vi "运维调试_五参数.vi"() -> ()   [LabVIEW 2016, in "斯坦道仪器.lvlib"]
uses:
  <vilib>/Utility/miscctls.llb/LVPointTypeDef.ctl
  PLC/PLC.lvlib
panel:
  in  "打开串口":bool
  in  "释放串口":bool
  in  "手动通电":bool
  out "多参数横条运行状态":T1(xcontrol)
  in  "数据区":i32(listbox)
  in  "探头选择":u16(ring)=9 items=["氨氮"=3, "水温"=9, "pH值"=10, "溶解氧"=11, "电导率"=12, "浊度"=13, "叶绿素a"=14, "藻密度"=15, "蓝绿藻"=16, "氧化还原电位"=17, "溶解氧%"=18, "盐度"=19]
  in  "测量数据区读取":bool
  in  "测量数据区":i32(listbox)
  in  "状态告警区读取":bool
  in  "状态告警区":i32(listbox)
  in  "自动校准":bool
  in  "读取KB":bool
  in  "写入KB":bool
  out "B":dbl caption="校准值B:"
  out "K":dbl caption="校准值K:"
  in  "校准区探头选择":u16(ring)=9 items=["氨氮"=3, "水温"=9, "pH值"=10, "溶解氧"=11, "电导率"=12, "浊度"=13, "叶绿素a"=14, "藻密度"=15, "蓝绿藻"=16, "氧化还原电位"=17, "溶解氧%"=18, "盐度"=19]
  in  "停止测量(单探)":bool
  in  "启动测量(单探)":bool
  in  "控制命令区探头选择":u16(ring)=9 items=["氨氮"=3, "水温"=9, "pH值"=10, "溶解氧"=11, "电导率"=12, "浊度"=13, "叶绿素a"=14, "藻密度"=15, "蓝绿藻"=16, "氧化还原电位"=17, "溶解氧%"=18, "盐度"=19]
  in  "同步时间":bool
  in  "初始化(清洗)":bool
  in  "停止测量(全部)":bool
  in  "启动测量(全部)":bool
  in  "关键参数区读取":bool
  in  "关键参数区":i32(listbox)
  in  "传感器参数读取":bool
  in  "传感器区":i32(listbox)
  in  "返回":bool
  in  "设置":bool
  out "运行状态":string
  out "开机状态":bool
  in  "停止":bool
  in  "手动启动":bool
  out "集成报警信息":string
  # "控制命令区"
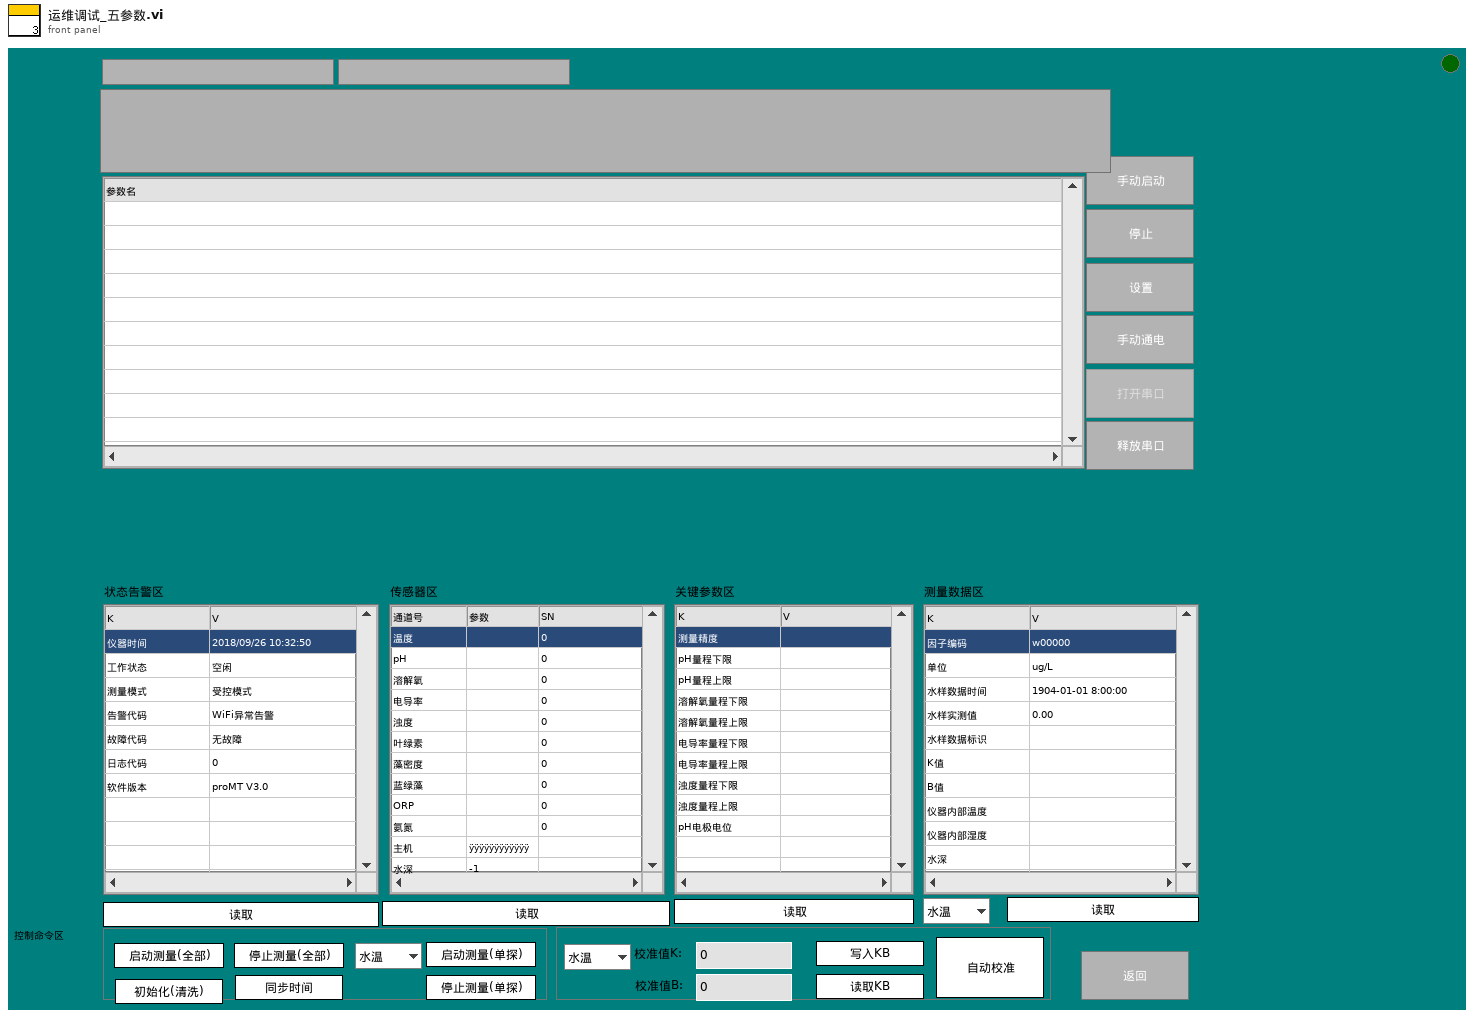
[diagram p1: front panel]
types:
  T1 = cluster{"系统时间":timestamp, "工作状态":u16, "测量模式":u16, "告警代码":enum16{"无告警", "缺试剂告警", "缺水样告警", "缺蒸馏水告警", "缺标液告警", "仪表漏液告警", "标定异常告警", "超量程告警", "加热异常", "低试剂预警", "超上限告警", "超下限告警", "仪表内部其他异常", "滴定异常告警", "电极异常告警", "量程切换告警", "参数设置告警", "PH电极电位异常", "电导率电极异常", "浊度光度异常", "溶解氧电极异常", "溶解氧光强异常", "温度异常告警", "PH异常告警", "溶解氧异常告警", "电导率异常告警", "浊度异常告警", "叶绿素异常告警", "藻密度异常告警", "蓝绿藻异常告警", "ORP异常告警", "氨氮异常告警", "清洁刷异常告警", "SD卡异常告警", "蓝牙异常告警", "Wifi异常告警", "流程异常告警"}, "故障代码":enum16{"无故障", "电机故障", "温度故障", "通讯故障", "滴定故障"}, "日志代码":u16, "软件版本":string}
  T2 = typedef "LVPointTypeDef.ctl" = cluster{"Horizontal":i16, "Vertical":i16}
  T3 = cluster{"时间标识":timestamp, "设备":string, "日志信息":string}
  T4 = enum16{"无告警", "缺试剂告警", "缺水样告警", "缺蒸馏水告警", "缺标液告警", "仪表漏液告警", "标定异常告警", "超量程告警", "加热异常", "低试剂预警", "超上限告警", "超下限告警", "仪表内部其他异常", "滴定异常告警", "电极异常告警", "量程切换告警", "参数设置告警", "PH电极电位异常", "电导率电极异常", "浊度光度异常", "溶解氧电极异常", "溶解氧光强异常", "温度异常告警", "PH异常告警", "溶解氧异常告警", "电导率异常告警", "浊度异常告警", "叶绿素异常告警", "藻密度异常告警", "蓝绿藻异常告警", "ORP异常告警", "氨氮异常告警", "清洁刷异常告警", "SD卡异常告警", "蓝牙异常告警", "Wifi异常告警", "流程异常告警"}
  T5 = cluster{"水温":dbl, "pH":dbl, "DO":dbl, "Cond":dbl, "Turb":dbl, "叶绿素":dbl, "藻密度":dbl, "蓝绿藻":dbl, "ORP":dbl, "NH3N":dbl}
  T6 = cluster{"因子编码":string, "单位":string, "标样参考值":sgl, "水样数据时间":timestamp, "水样实测值":sgl, "水样数据标识":string, "K":sgl, "B":sgl, "T":sgl, "H":sgl, "水深":sgl}
  T7 = enum8{"Enabled", "Disabled", "Disabled and Grayed Out"}
  T8 = cluster{"测量模式":enum16{"待机", "水样测试", "标样核查", "零点核查", "跨度核查", "空白测试", "平行样测试", "加标回收", "空白校准", "标样校准", "初始化（清洗）"}, "数据标记表":string, "测量时间":dbl}
  T9 = cluster{"starting address":u16, "holding register value":u16}
  T10 = enum16{"idle", "init", "读状态", "读参数", "多个写入", "单个写入", "线圈写入"}
  T11 = enum32{"Bad", "Idle", "Run top level", "Running"}
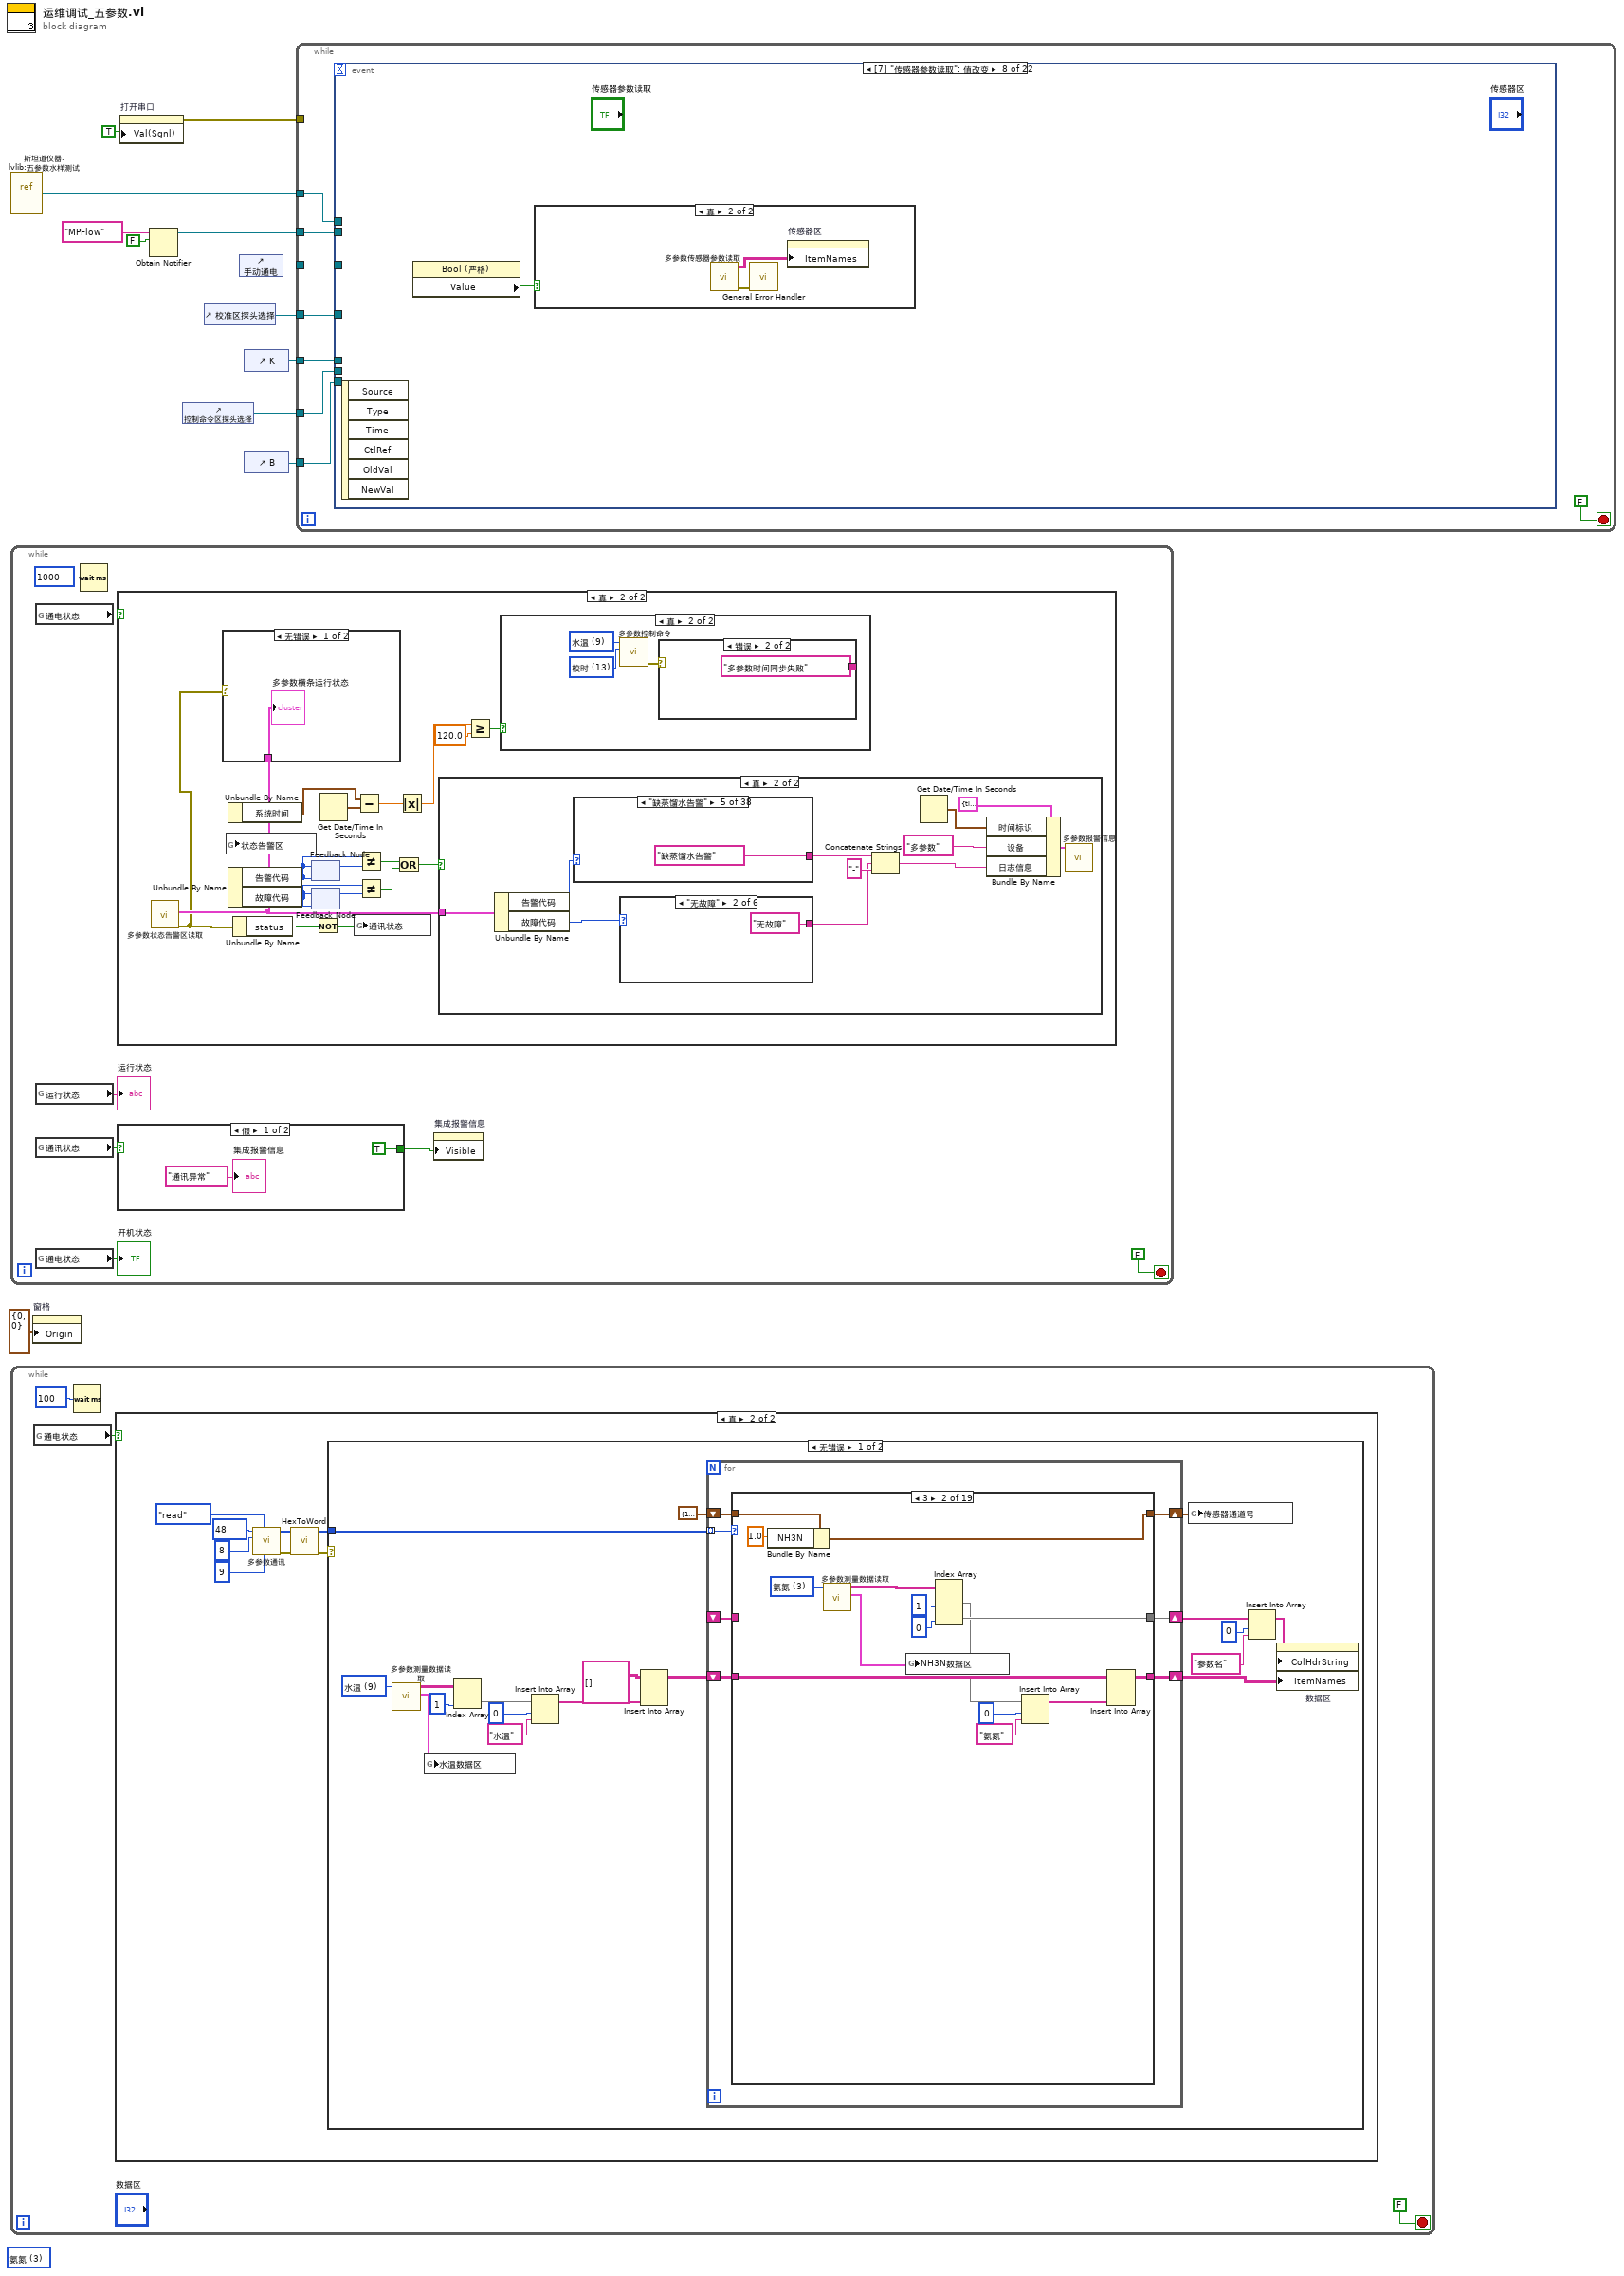
[diagram p0: block diagram]
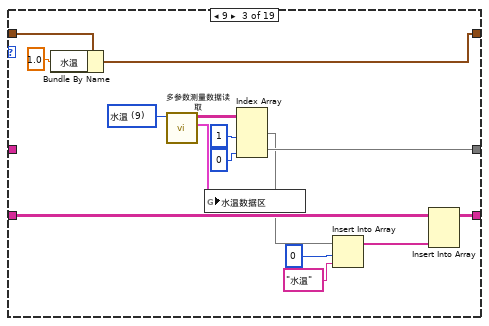
[diagram p4: hidden frame]
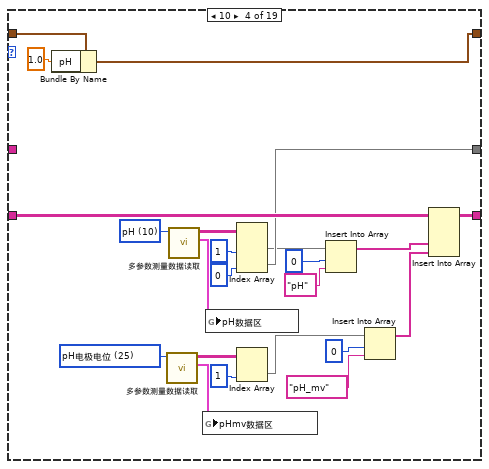
[diagram p5: hidden frame]
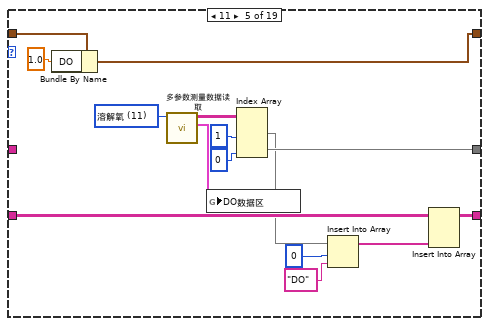
[diagram p6: hidden frame]
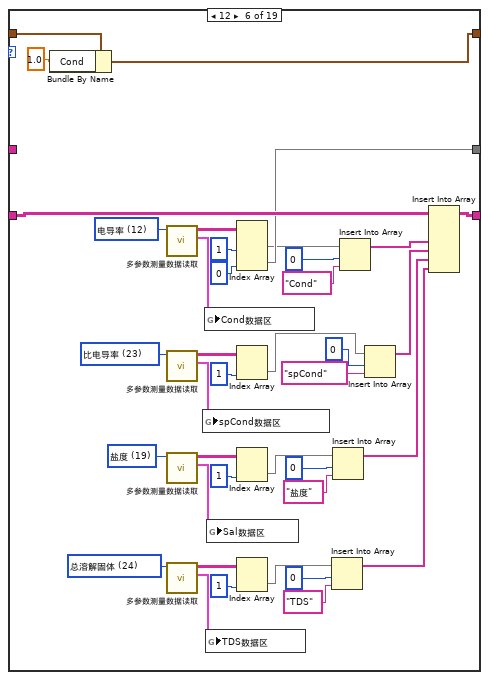
[diagram p7: hidden frame]
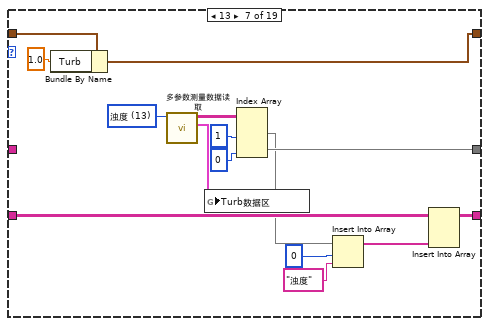
[diagram p8: hidden frame]
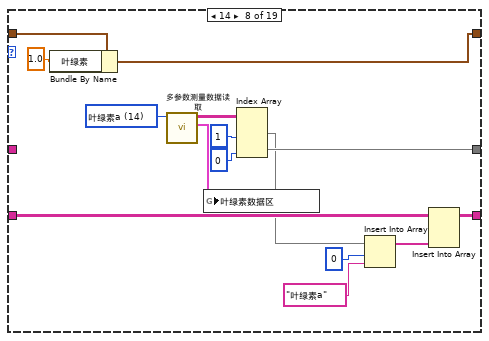
[diagram p9: hidden frame]
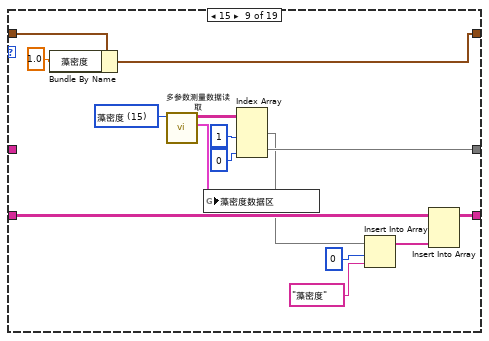
[diagram p10: hidden frame]
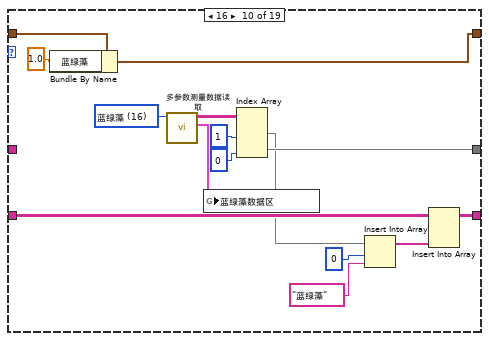
[diagram p11: hidden frame]
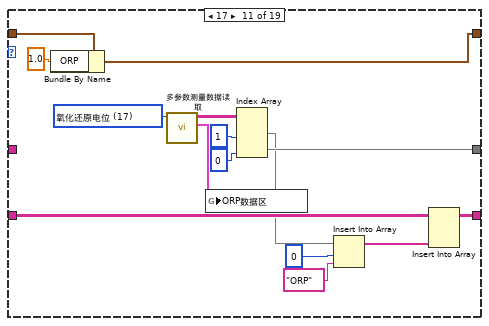
[diagram p12: hidden frame]
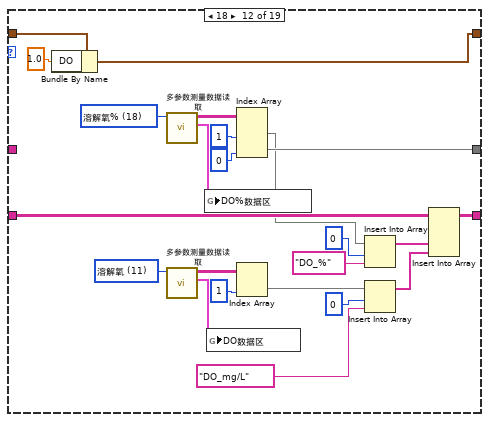
[diagram p13: hidden frame]
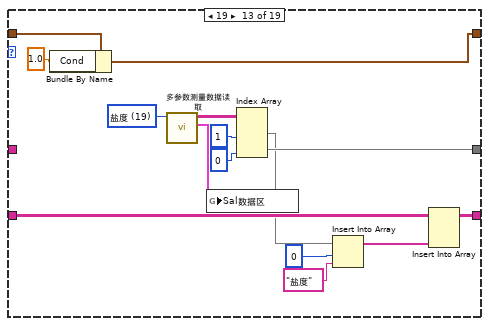
[diagram p14: hidden frame]
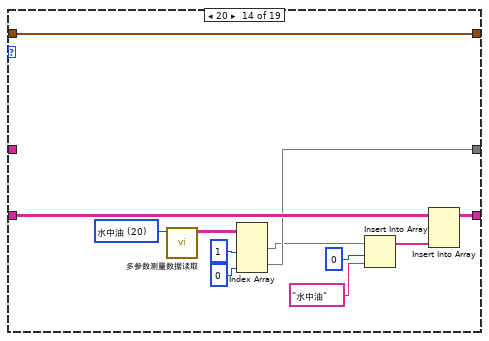
[diagram p15: hidden frame]
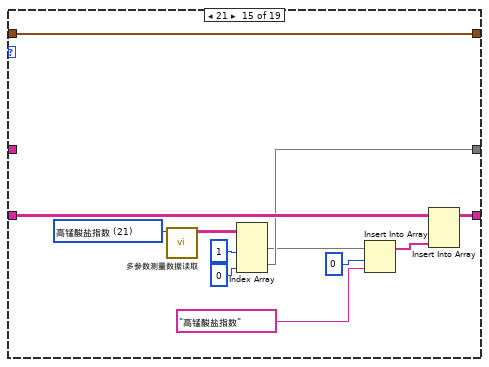
[diagram p16: hidden frame]
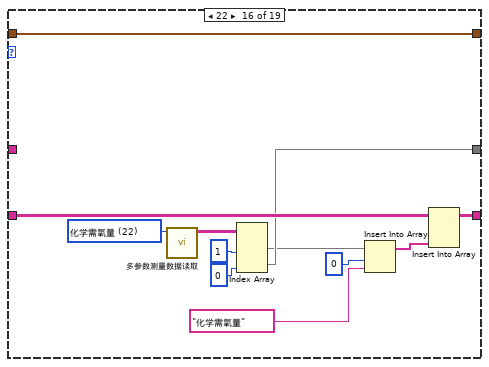
[diagram p17: hidden frame]
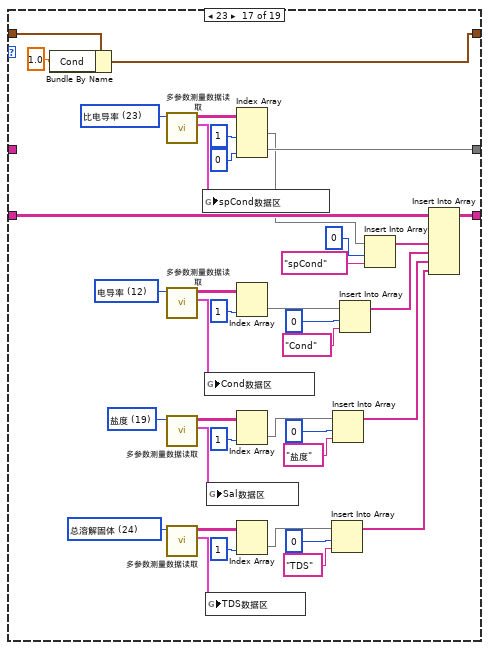
[diagram p18: hidden frame]
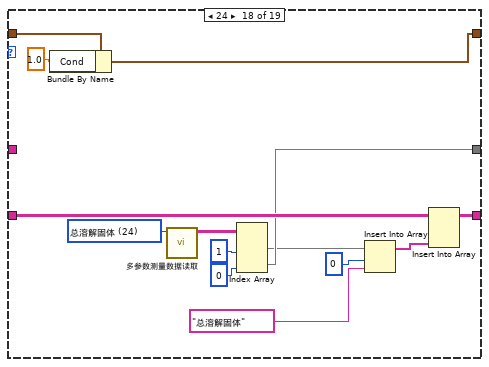
[diagram p19: hidden frame]
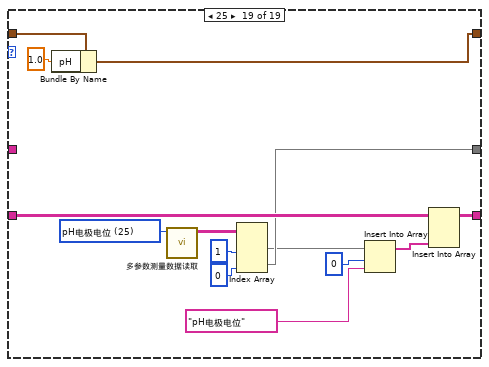
[diagram p20: hidden frame]
diagram:
  (unwired) u16 3 items=["氨氮"=3, "水温"=9, "pH"=10, "溶解氧"=11, "电导率"=12, "浊度"=13, "叶绿素a"=14, "藻密度"=15, "蓝绿藻"=16, "氧化还原电位"=17, "溶解氧%"=18, "盐度"=19, "水中油"=20, "高锰酸盐指数"=21, "化学需氧量"=22, "比电导率"=23, "总溶解固体"=24, "pH电极电位"=25] ("下拉列表")
  n1 = vi-ref "斯坦道仪器.lvlib:五参数水样测试.vi"() -> (w9:refnum<vi>)
  n2 = while {
    stop <- FALSE stop-if-true
    n3 = global read "多参数全局变量.vi" "通电状态"() -> (w13:bool)
    n4 = global read "多参数全局变量.vi" "运行状态"() -> (→"运行状态":string)
    n5 = global read "多参数全局变量.vi" "通讯状态"() -> (w17:bool)
    n6 = global read "多参数全局变量.vi" "通电状态"() -> (→"开机状态":bool)
    n7 = Wait (ms)(milliseconds to wait=u32 1000 ("等待时间（毫秒）")) -> ()  [unwired: 1 out]
    n8 = case shown="真" w13 {
      frame False {
      }
      frame True {
        n9 = call "多参数状态告警区读取.vi"() -> ("error out"=w20:errorcluster, "状态告警块"=w27:T1)  [unwired: 9 in, 1 out]
        n10 = case shown="无错误" w20 {
          tunnel: w27 -> [w37 _]
          frame No Error {
            "多参数横条运行状态" <- w37
          }
          frame Error {
          }
        }
        n11 = global write "多参数全局变量.vi" "状态告警区"(w27) -> ()
        n12 = Unbundle By Name(w27) -> ("系统时间"=w26:timestamp)
        n13 = Unbundle By Name(w27) -> ("告警代码"=w35:T4, "故障代码"=w33:enum16{"无故障", "电机故障", "温度故障", "通讯故障", "滴定故障"})
        n14 = Unbundle By Name(w20) -> ("status"=w29:bool)
        n15 = feedback #1(w35) -> (w36:T4)
        n16 = feedback-in #1(w35) -> ()
        n17 = feedback #2(w33) -> (w34:enum16{"无故障", "电机故障", "温度故障", "通讯故障", "滴定故障"})
        n18 = feedback-in #2(w33) -> ()
        n19 = Not(x=w29) -> (.not. x?=w28:bool)
        n20 = Get Date/Time In Seconds() -> (seconds since 1Jan1904=w25:timestamp)
        n21 = global write "多参数全局变量.vi" "通讯状态"(w28) -> ()
        n22 = Subtract(x=w26, y=w25) -> (x-y=w24:dbl)
        n23 = Not Equal?(x=w35, y=w36) -> (x != y?=w31:bool)
        n24 = Not Equal?(x=w33, y=w34) -> (x != y?=w32:bool)
        n25 = Or(x=w31, y=w32) -> (x .or. y?=w30:bool)
        n26 = Absolute Value(x=w24) -> (abs(x)=w23:dbl)
        n27 = case shown="真" w30 {
          tunnel: w27 -> [_ w53]
          frame False {
          }
          frame True {
            n28 = Unbundle By Name(w53) -> ("告警代码"=w52:T4, "故障代码"=w51:enum16{"无故障", "电机故障", "温度故障", "通讯故障", "滴定故障"})
            n29 = case shown="\"缺蒸馏水告警\"" w52 {
              selector: w52 -> [w64 _ _ _ _ _ _ _ _ _ _ _ _ _ _ _ _ _ _ _ _ _ _ _ _ _ _ _ _ _ _ _ _ _ _ _ _ _]
              tunnel: [w63 "无告警" "缺试剂告警" "缺水样告警" "缺蒸馏水告警" "缺标液告警" "仪表漏液告警" "标定异常告警" "超量程告警" "加热异常" "低试剂预警" "超上限告警" "超下限告警" "仪表内部其他异常" "滴定异常告警" "电极异常告警" "量程切换告警" "参数设置告警" "PH电极电位异常" "电导率电极异常" "浊度光度异常" "溶解氧电极异常" "溶解氧光强异常" "温度异常告警" "PH异常告警" "溶解氧异常告警" "电导率异常告警" "浊度异常告警" "叶绿素异常告警" "藻密度异常告警" "蓝绿藻异常告警" "ORP异常告警" "氨氮异常告警" "清洁刷异常告警" "SD卡异常告警" "蓝牙异常告警" "WiFi异常告警" "流程异常告警"] -> w50
              frame Default {
                n30 = Format Into String(format string="%d" ("格式字符串"), initial string="未知" ("工作状态"), w64) -> (resulting string=w63:string)  [unwired: 1 in, 1 out]
              }
              frame "无告警" {
              }
              frame "缺试剂告警" {
              }
              frame "缺水样告警" {
              }
              frame "缺蒸馏水告警" {
              }
              frame "缺标液告警" {
              }
              frame "仪表漏液告警" {
              }
              frame "标定异常告警" {
              }
              frame "超量程告警" {
              }
              frame "加热异常" {
              }
              frame "低试剂预警" {
              }
              frame "超上限告警" {
              }
              frame "超下限告警" {
              }
              frame "仪表内部其他异常" {
              }
              frame "滴定异常告警" {
              }
              frame "电极异常告警" {
              }
              frame "量程切换告警" {
              }
              frame "参数设置告警" {
              }
              frame "PH电极电位异常" {
              }
              frame "电导率电极异常" {
              }
              frame "浊度光度异常" {
              }
              frame "溶解氧电极异常" {
              }
              frame "溶解氧光强异常" {
              }
              frame "温度异常告警" {
              }
              frame "PH异常告警" {
              }
              frame "溶解氧异常告警" {
              }
              frame "电导率异常告警" {
              }
              frame "浊度异常告警" {
              }
              frame "叶绿素异常告警" {
              }
              frame "藻密度异常告警" {
              }
              frame "蓝绿藻异常告警" {
              }
              frame "ORP异常告警" {
              }
              frame "氨氮异常告警" {
              }
              frame "清洁刷异常告警" {
              }
              frame "SD卡异常告警" {
              }
              frame "蓝牙异常告警" {
              }
              frame "Wifi异常告警" {
              }
              frame "流程异常告警" {
              }
            }
            n31 = case shown="\"无故障\"" w51 {
              selector: w51 -> [w55 _ _ _ _ _]
              tunnel: [w54 "无故障" "电机故障" "温度故障" "通讯故障" "滴定故障"] -> w49
              frame Default {
                n32 = Format Into String(format string="%d" ("格式字符串"), initial string="未知" ("工作状态"), w55) -> (resulting string=w54:string)  [unwired: 1 in, 1 out]
              }
              frame "无故障" {
              }
              frame "电机故障" {
              }
              frame "温度故障" {
              }
              frame "通讯故障" {
              }
              frame "滴定故障" {
              }
            }
            n33 = Concatenate Strings(w50, "-" ("字符串"), w49) -> (w45:string)
            n34 = Get Date/Time In Seconds() -> (seconds since 1Jan1904=w44:timestamp)
            n35 = Bundle By Name(cluster=T3 {"时间标识"=timestamp(0 s since 1904-01-01), "设备"="", "日志信息"=""} ("data in"), "时间标识"=w44, "设备"="多参数", "日志信息"=w45) -> (w46:T3)
            n36 = call "多参数报警信息.vi"("data in"=w46) -> ()  [unwired: 10 in, 1 out]
          }
        }
        n37 = Greater Or Equal?(x=w23, y=120.0) -> (x >= y?=w22:bool)
        n38 = case shown="真" w22 {
          frame False {
          }
          frame True {
            w38 = u16 13 items=["启动测量（全部）"=1, "初始化（清洗）"=10, "停止测量（全部）"=11, "校时"=13, "启动测量（单个传感器）"=19, "停止测量（单个传感器）"=20] ("控制命令")
            w39 = u16 9 items=["氨氮"=3, "水温"=9, "pH值"=10, "溶解氧"=11, "电导率"=12, "浊度"=13, "叶绿素a"=14, "藻密度"=15, "蓝绿藻"=16, "氧化还原电位"=17, "溶解氧%"=18, "盐度"=19] ("站号")
            n39 = call "多参数控制命令.vi"("控制命令"=w38, "站号"=w39) -> ("error out"=w40:errorcluster)  [unwired: 9 in]
            n40 = case shown="错误" w40 {
              tunnel: ["多参数时间同步成功" ("消息") "多参数时间同步失败" ("消息")] -> _
              frame No Error {
              }
              frame Error {
              }
            }
          }
        }
      }
    }
    n41 = case shown="假" w17 {
      tunnel: [TRUE ("可见") _] -> w16
      frame False {
        "集成报警信息" <- "通讯异常" ("集成报警信息")
      }
      frame True {
      }
    }
    n42 = property on="集成报警信息" class="Str"("Visible"=w16) -> ()  [unwired: 2 in, 2 out]
  }
  n43 = while {
    stop <- FALSE stop-if-true
    n44 = global read "多参数全局变量.vi" "通电状态"() -> (w106:bool)
    n45 = Wait (ms)(milliseconds to wait=u32 100 ("等待时间（毫秒）")) -> ()  [unwired: 1 out]
    n46 = case shown="真" w106 {
      frame False {
      }
      frame True {
        n47 = call "多参数通讯.vi"("Slave ID"=u8 9, "STEP"=enum16{"open", "read", "write", "close"}."read", "quantity"=u16 8, "starting address"=u16 48) -> ("error out"=w111:errorcluster, "Registers"=w112:u16[])  [unwired: 5 in, 1 out]
        n48 = call "HexToWord.vi"("数组"=w112) -> ("WORD"=w115:u16[])  [unwired: 10 in]
        n49 = case shown="无错误" w111 {
          tunnel: w115 -> [w130 _]
          frame No Error {
            w127 = u16 9 items=["氨氮"=3, "水温"=9, "pH"=10, "溶解氧"=11, "电导率"=12, "浊度"=13, "叶绿素a"=14, "藻密度"=15, "蓝绿藻"=16, "氧化还原电位"=17, "溶解氧%"=18, "盐度"=19, "水中油"=20, "高锰酸盐指数"=21, "化学需氧量"=22, "比电导率"=23, "总溶解固体"=24, "pH电极电位"=25] ("下拉列表")
            n50 = call "多参数测量数据读取.vi"("探头选择"=w127) -> ("测量数据块"=w116:T6, "添加的数组"=w126:string[][])  [unwired: 8 in, 1 out]
            n51 = global write "多参数全局变量.vi" "水温数据区"(w116) -> ()
            n52 = Index Array(array=w126, index (col)=1 ("禁用的索引 (列)")) -> (element=w121:string[])  [unwired: 1 in]
            n53 = Insert Into Array(array=w121, index=0 ("索引"), new element="水温") -> (w123:string[])
            n54 = Insert Into Array(array=string[][] [] ("子数组"), new element=w123) -> (w119:string[][])  [unwired: 2 in]
            n55 = for {
              tunnel: w130 -> [w140] mode=indexing
              shift-right: [w138] -> w128
              shift-left: w119 -> [w139]
              shift-right: [w137] -> w129
              shift-left: _ -> [w136]
              shift-right: [w135] -> w117
              shift-left: T5 {"水温"=1.0, "pH"=0.0, "DO"=0.0, "Cond"=0.0, "Turb"=0.0, "叶绿素"=0.0, "藻密度"=0.0, "蓝绿藻"=0.0, "ORP"=0.0, "NH3N"=0.0} ("传感器通道号") -> [w134]
              n56 = case shown="3" w140 {
                tunnel: w139 -> [w143 w154 w169 w192 w207 w246 w261 w276 w291 w306 w321 w344 w359 w371 w383 w395 w434 w448 w462]
                tunnel: [w143 w153 w168 w191 w206 w245 w260 w275 w290 w305 w320 w343 w358 w370 w382 w394 w433 w447 w461] -> w138
                tunnel: [w142 w151 w166 w189 w204 w243 w258 w273 w288 w303 w318 w341 w356 w368 w380 w392 w431 w445 w459] -> w137
                tunnel: w136 -> [w142 _ _ _ _ _ _ _ _ _ _ _ _ _ _ _ _ _ _]
                tunnel: [w141 w145 w160 w176 w198 w216 w252 w267 w282 w297 w312 w328 w350 w364 w376 w388 w425 w439 w453] -> w135
                tunnel: w134 -> [w141 w147 w162 w178 w200 w217 w253 w268 w283 w298 w313 w329 w351 w364 w376 w388 w426 w440 w454]
                frame 0, Default {
                }
                frame 3 {
                  w158 = u16 3 items=["氨氮"=3, "水温"=9, "pH"=10, "溶解氧"=11, "电导率"=12, "浊度"=13, "叶绿素a"=14, "藻密度"=15, "蓝绿藻"=16, "氧化还原电位"=17, "溶解氧%"=18, "盐度"=19, "水中油"=20, "高锰酸盐指数"=21, "化学需氧量"=22, "比电导率"=23, "总溶解固体"=24, "pH电极电位"=25] ("下拉列表")
                  n57 = Bundle By Name(cluster=w147, "NH3N"=1.0) -> (w145:T5)
                  n58 = call "多参数测量数据读取.vi"("探头选择"=w158) -> ("测量数据块"=w144:T6, "添加的数组"=w157:string[][])  [unwired: 8 in, 1 out]
                  n59 = global write "多参数全局变量.vi" "NH3N数据区"(w144) -> ()
                  n60 = Index Array(array=w157, index (col) #1=1 ("禁用的索引 (列)"), index (col) #2=0 ("禁用的索引 (列)")) -> (element #1=w148:string[], element #2=w151:string[])  [unwired: 2 in]
                  n61 = Insert Into Array(array=w148, index=0 ("索引"), new element="氨氮") -> (w152:string[])
                  n62 = Insert Into Array(array=w154, new element=w152) -> (w153:string[][])  [unwired: 2 in]
                }
                frame 9 {
                  w173 = u16 9 items=["氨氮"=3, "水温"=9, "pH"=10, "溶解氧"=11, "电导率"=12, "浊度"=13, "叶绿素a"=14, "藻密度"=15, "蓝绿藻"=16, "氧化还原电位"=17, "溶解氧%"=18, "盐度"=19, "水中油"=20, "高锰酸盐指数"=21, "化学需氧量"=22, "比电导率"=23, "总溶解固体"=24, "pH电极电位"=25] ("下拉列表")
                  n63 = Bundle By Name(cluster=w162, "水温"=1.0) -> (w160:T5)
                  n64 = call "多参数测量数据读取.vi"("探头选择"=w173) -> ("测量数据块"=w159:T6, "添加的数组"=w172:string[][])  [unwired: 8 in, 1 out]
                  n65 = global write "多参数全局变量.vi" "水温数据区"(w159) -> ()
                  n66 = Index Array(array=w172, index (col) #1=1 ("禁用的索引 (列)"), index (col) #2=0 ("禁用的索引 (列)")) -> (element #1=w163:string[], element #2=w166:string[])  [unwired: 2 in]
                  n67 = Insert Into Array(array=w163, index=0 ("索引"), new element="水温") -> (w167:string[])
                  n68 = Insert Into Array(array=w169, new element=w167) -> (w168:string[][])  [unwired: 2 in]
                }
                frame 10 {
                  w180 = u16 25 items=["氨氮"=3, "水温"=9, "pH"=10, "溶解氧"=11, "电导率"=12, "浊度"=13, "叶绿素a"=14, "藻密度"=15, "蓝绿藻"=16, "氧化还原电位"=17, "溶解氧%"=18, "盐度"=19, "水中油"=20, "高锰酸盐指数"=21, "化学需氧量"=22, "比电导率"=23, "总溶解固体"=24, "pH电极电位"=25] ("下拉列表")
                  w196 = u16 10 items=["氨氮"=3, "水温"=9, "pH"=10, "溶解氧"=11, "电导率"=12, "浊度"=13, "叶绿素a"=14, "藻密度"=15, "蓝绿藻"=16, "氧化还原电位"=17, "溶解氧%"=18, "盐度"=19, "水中油"=20, "高锰酸盐指数"=21, "化学需氧量"=22, "比电导率"=23, "总溶解固体"=24, "pH电极电位"=25] ("下拉列表")
                  n69 = Bundle By Name(cluster=w178, "pH"=1.0) -> (w176:T5)
                  n70 = call "多参数测量数据读取.vi"("探头选择"=w180) -> ("测量数据块"=w174:T6, "添加的数组"=w181:string[][])  [unwired: 8 in, 1 out]
                  n71 = call "多参数测量数据读取.vi"("探头选择"=w196) -> ("测量数据块"=w175:T6, "添加的数组"=w195:string[][])  [unwired: 8 in, 1 out]
                  n72 = global write "多参数全局变量.vi" "pHmv数据区"(w174) -> ()
                  n73 = global write "多参数全局变量.vi" "pH数据区"(w175) -> ()
                  n74 = Index Array(array=w195, index (col) #1=1 ("禁用的索引 (列)"), index (col) #2=0 ("禁用的索引 (列)")) -> (element #1=w186:string[], element #2=w189:string[])  [unwired: 2 in]
                  n75 = Index Array(array=w181, index (col)=1 ("禁用的索引 (列)")) -> (element=w185:string[])  [unwired: 1 in]
                  n76 = Insert Into Array(array=w186, index=0 ("索引"), new element="pH") -> (w190:string[])
                  n77 = Insert Into Array(array=w185, index=0 ("索引"), new element="pH_mv") -> (w179:string[])
                  n78 = Insert Into Array(array=w192, new element #1=w190, new element #2=w179) -> (w191:string[][])  [unwired: 2 in]
                }
                frame 11 {
                  w211 = u16 11 items=["氨氮"=3, "水温"=9, "pH"=10, "溶解氧"=11, "电导率"=12, "浊度"=13, "叶绿素a"=14, "藻密度"=15, "蓝绿藻"=16, "氧化还原电位"=17, "溶解氧%"=18, "盐度"=19, "水中油"=20, "高锰酸盐指数"=21, "化学需氧量"=22, "比电导率"=23, "总溶解固体"=24, "pH电极电位"=25] ("下拉列表")
                  n79 = Bundle By Name(cluster=w200, "DO"=1.0) -> (w198:T5)
                  n80 = call "多参数测量数据读取.vi"("探头选择"=w211) -> ("测量数据块"=w197:T6, "添加的数组"=w210:string[][])  [unwired: 8 in, 1 out]
                  n81 = global write "多参数全局变量.vi" "DO数据区"(w197) -> ()
                  n82 = Index Array(array=w210, index (col) #1=1 ("禁用的索引 (列)"), index (col) #2=0 ("禁用的索引 (列)")) -> (element #1=w201:string[], element #2=w204:string[])  [unwired: 2 in]
                  n83 = Insert Into Array(array=w201, index=0 ("索引"), new element="DO") -> (w205:string[])
                  n84 = Insert Into Array(array=w207, new element=w205) -> (w206:string[][])  [unwired: 2 in]
                }
                frame 12 {
                  w220 = u16 24 items=["氨氮"=3, "水温"=9, "pH"=10, "溶解氧"=11, "电导率"=12, "浊度"=13, "叶绿素a"=14, "藻密度"=15, "蓝绿藻"=16, "氧化还原电位"=17, "溶解氧%"=18, "盐度"=19, "水中油"=20, "高锰酸盐指数"=21, "化学需氧量"=22, "比电导率"=23, "总溶解固体"=24, "pH电极电位"=25] ("下拉列表")
                  w232 = u16 19 items=["氨氮"=3, "水温"=9, "pH"=10, "溶解氧"=11, "电导率"=12, "浊度"=13, "叶绿素a"=14, "藻密度"=15, "蓝绿藻"=16, "氧化还原电位"=17, "溶解氧%"=18, "盐度"=19, "水中油"=20, "高锰酸盐指数"=21, "化学需氧量"=22, "比电导率"=23, "总溶解固体"=24, "pH电极电位"=25] ("下拉列表")
                  w234 = u16 23 items=["氨氮"=3, "水温"=9, "pH"=10, "溶解氧"=11, "电导率"=12, "浊度"=13, "叶绿素a"=14, "藻密度"=15, "蓝绿藻"=16, "氧化还原电位"=17, "溶解氧%"=18, "盐度"=19, "水中油"=20, "高锰酸盐指数"=21, "化学需氧量"=22, "比电导率"=23, "总溶解固体"=24, "pH电极电位"=25] ("下拉列表")
                  w250 = u16 12 items=["氨氮"=3, "水温"=9, "pH"=10, "溶解氧"=11, "电导率"=12, "浊度"=13, "叶绿素a"=14, "藻密度"=15, "蓝绿藻"=16, "氧化还原电位"=17, "溶解氧%"=18, "盐度"=19, "水中油"=20, "高锰酸盐指数"=21, "化学需氧量"=22, "比电导率"=23, "总溶解固体"=24, "pH电极电位"=25] ("下拉列表")
                  n85 = Bundle By Name(cluster=w217, "Cond"=1.0 ("DO")) -> (w216:T5)
                  n86 = call "多参数测量数据读取.vi"("探头选择"=w250) -> ("测量数据块"=w215:T6, "添加的数组"=w249:string[][])  [unwired: 8 in, 1 out]
                  n87 = call "多参数测量数据读取.vi"("探头选择"=w234) -> ("测量数据块"=w213:T6, "添加的数组"=w235:string[][])  [unwired: 8 in, 1 out]
                  n88 = call "多参数测量数据读取.vi"("探头选择"=w232) -> ("测量数据块"=w214:T6, "添加的数组"=w231:string[][])  [unwired: 8 in, 1 out]
                  n89 = call "多参数测量数据读取.vi"("探头选择"=w220) -> ("测量数据块"=w212:T6, "添加的数组"=w221:string[][])  [unwired: 8 in, 1 out]
                  n90 = global write "多参数全局变量.vi" "spCond数据区"(w213) -> ()
                  n91 = global write "多参数全局变量.vi" "Cond数据区"(w215) -> ()
                  n92 = global write "多参数全局变量.vi" "TDS数据区"(w212) -> ()
                  n93 = global write "多参数全局变量.vi" "Sal数据区"(w214) -> ()
                  n94 = Index Array(array=w249, index (col) #1=1 ("禁用的索引 (列)"), index (col) #2=0 ("禁用的索引 (列)")) -> (element #1=w240:string[], element #2=w243:string[])  [unwired: 2 in]
                  n95 = Index Array(array=w235, index (col)=1 ("禁用的索引 (列)")) -> (element=w239:string[])  [unwired: 1 in]
                  n96 = Index Array(array=w231, index (col)=1 ("禁用的索引 (列)")) -> (element=w227:string[])  [unwired: 1 in]
                  n97 = Index Array(array=w221, index (col)=1 ("禁用的索引 (列)")) -> (element=w225:string[])  [unwired: 1 in]
                  n98 = Insert Into Array(array=w225, index=0 ("索引"), new element="TDS") -> (w219:string[])
                  n99 = Insert Into Array(array=w227, index=0 ("索引"), new element="盐度") -> (w226:string[])
                  n100 = Insert Into Array(array=w240, index=0 ("索引"), new element="Cond") -> (w244:string[])
                  n101 = Insert Into Array(array=w239, index=0 ("索引"), new element="spCond") -> (w233:string[])
                  n102 = Insert Into Array(array=w246, new element #1=w244, new element #2=w233, new element #3=w226, new element #4=w219) -> (w245:string[][])  [unwired: 2 in]
                }
                frame 13 {
                  w265 = u16 13 items=["氨氮"=3, "水温"=9, "pH"=10, "溶解氧"=11, "电导率"=12, "浊度"=13, "叶绿素a"=14, "藻密度"=15, "蓝绿藻"=16, "氧化还原电位"=17, "溶解氧%"=18, "盐度"=19, "水中油"=20, "高锰酸盐指数"=21, "化学需氧量"=22, "比电导率"=23, "总溶解固体"=24, "pH电极电位"=25] ("下拉列表")
                  n103 = Bundle By Name(cluster=w253, "Turb"=1.0 ("DO")) -> (w252:T5)
                  n104 = call "多参数测量数据读取.vi"("探头选择"=w265) -> ("测量数据块"=w251:T6, "添加的数组"=w264:string[][])  [unwired: 8 in, 1 out]
                  n105 = global write "多参数全局变量.vi" "Turb数据区"(w251) -> ()
                  n106 = Index Array(array=w264, index (col) #1=1 ("禁用的索引 (列)"), index (col) #2=0 ("禁用的索引 (列)")) -> (element #1=w255:string[], element #2=w258:string[])  [unwired: 2 in]
                  n107 = Insert Into Array(array=w255, index=0 ("索引"), new element="浊度") -> (w259:string[])
                  n108 = Insert Into Array(array=w261, new element=w259) -> (w260:string[][])  [unwired: 2 in]
                }
                frame 14 {
                  w280 = u16 14 items=["氨氮"=3, "水温"=9, "pH"=10, "溶解氧"=11, "电导率"=12, "浊度"=13, "叶绿素a"=14, "藻密度"=15, "蓝绿藻"=16, "氧化还原电位"=17, "溶解氧%"=18, "盐度"=19, "水中油"=20, "高锰酸盐指数"=21, "化学需氧量"=22, "比电导率"=23, "总溶解固体"=24, "pH电极电位"=25] ("下拉列表")
                  n109 = Bundle By Name(cluster=w268, "叶绿素"=1.0 ("DO")) -> (w267:T5)
                  n110 = call "多参数测量数据读取.vi"("探头选择"=w280) -> ("测量数据块"=w266:T6, "添加的数组"=w279:string[][])  [unwired: 8 in, 1 out]
                  n111 = global write "多参数全局变量.vi" "叶绿素数据区"(w266) -> ()
                  n112 = Index Array(array=w279, index (col) #1=1 ("禁用的索引 (列)"), index (col) #2=0 ("禁用的索引 (列)")) -> (element #1=w270:string[], element #2=w273:string[])  [unwired: 2 in]
                  n113 = Insert Into Array(array=w270, index=0 ("索引"), new element="叶绿素a") -> (w274:string[])
                  n114 = Insert Into Array(array=w276, new element=w274) -> (w275:string[][])  [unwired: 2 in]
                }
                frame 15 {
                  w295 = u16 15 items=["氨氮"=3, "水温"=9, "pH"=10, "溶解氧"=11, "电导率"=12, "浊度"=13, "叶绿素a"=14, "藻密度"=15, "蓝绿藻"=16, "氧化还原电位"=17, "溶解氧%"=18, "盐度"=19, "水中油"=20, "高锰酸盐指数"=21, "化学需氧量"=22, "比电导率"=23, "总溶解固体"=24, "pH电极电位"=25] ("下拉列表")
                  n115 = Bundle By Name(cluster=w283, "藻密度"=1.0 ("DO")) -> (w282:T5)
                  n116 = call "多参数测量数据读取.vi"("探头选择"=w295) -> ("测量数据块"=w281:T6, "添加的数组"=w294:string[][])  [unwired: 8 in, 1 out]
                  n117 = global write "多参数全局变量.vi" "藻密度数据区"(w281) -> ()
                  n118 = Index Array(array=w294, index (col) #1=1 ("禁用的索引 (列)"), index (col) #2=0 ("禁用的索引 (列)")) -> (element #1=w285:string[], element #2=w288:string[])  [unwired: 2 in]
                  n119 = Insert Into Array(array=w285, index=0 ("索引"), new element="藻密度") -> (w289:string[])
                  n120 = Insert Into Array(array=w291, new element=w289) -> (w290:string[][])  [unwired: 2 in]
                }
                frame 16 {
                  w310 = u16 16 items=["氨氮"=3, "水温"=9, "pH"=10, "溶解氧"=11, "电导率"=12, "浊度"=13, "叶绿素a"=14, "藻密度"=15, "蓝绿藻"=16, "氧化还原电位"=17, "溶解氧%"=18, "盐度"=19, "水中油"=20, "高锰酸盐指数"=21, "化学需氧量"=22, "比电导率"=23, "总溶解固体"=24, "pH电极电位"=25] ("下拉列表")
                  n121 = Bundle By Name(cluster=w298, "蓝绿藻"=1.0 ("DO")) -> (w297:T5)
                  n122 = call "多参数测量数据读取.vi"("探头选择"=w310) -> ("测量数据块"=w296:T6, "添加的数组"=w309:string[][])  [unwired: 8 in, 1 out]
                  n123 = global write "多参数全局变量.vi" "蓝绿藻数据区"(w296) -> ()
                  n124 = Index Array(array=w309, index (col) #1=1 ("禁用的索引 (列)"), index (col) #2=0 ("禁用的索引 (列)")) -> (element #1=w300:string[], element #2=w303:string[])  [unwired: 2 in]
                  n125 = Insert Into Array(array=w300, index=0 ("索引"), new element="蓝绿藻") -> (w304:string[])
                  n126 = Insert Into Array(array=w306, new element=w304) -> (w305:string[][])  [unwired: 2 in]
                }
                frame 17 {
                  w325 = u16 17 items=["氨氮"=3, "水温"=9, "pH"=10, "溶解氧"=11, "电导率"=12, "浊度"=13, "叶绿素a"=14, "藻密度"=15, "蓝绿藻"=16, "氧化还原电位"=17, "溶解氧%"=18, "盐度"=19, "水中油"=20, "高锰酸盐指数"=21, "化学需氧量"=22, "比电导率"=23, "总溶解固体"=24, "pH电极电位"=25] ("下拉列表")
                  n127 = Bundle By Name(cluster=w313, "ORP"=1.0 ("DO")) -> (w312:T5)
                  n128 = call "多参数测量数据读取.vi"("探头选择"=w325) -> ("测量数据块"=w311:T6, "添加的数组"=w324:string[][])  [unwired: 8 in, 1 out]
                  n129 = global write "多参数全局变量.vi" "ORP数据区"(w311) -> ()
                  n130 = Index Array(array=w324, index (col) #1=1 ("禁用的索引 (列)"), index (col) #2=0 ("禁用的索引 (列)")) -> (element #1=w315:string[], element #2=w318:string[])  [unwired: 2 in]
                  n131 = Insert Into Array(array=w315, index=0 ("索引"), new element="ORP") -> (w319:string[])
                  n132 = Insert Into Array(array=w321, new element=w319) -> (w320:string[][])  [unwired: 2 in]
                }
                frame 18 {
                  w332 = u16 11 items=["氨氮"=3, "水温"=9, "pH"=10, "溶解氧"=11, "电导率"=12, "浊度"=13, "叶绿素a"=14, "藻密度"=15, "蓝绿藻"=16, "氧化还原电位"=17, "溶解氧%"=18, "盐度"=19, "水中油"=20, "高锰酸盐指数"=21, "化学需氧量"=22, "比电导率"=23, "总溶解固体"=24, "pH电极电位"=25] ("下拉列表")
                  w348 = u16 18 items=["氨氮"=3, "水温"=9, "pH"=10, "溶解氧"=11, "电导率"=12, "浊度"=13, "叶绿素a"=14, "藻密度"=15, "蓝绿藻"=16, "氧化还原电位"=17, "溶解氧%"=18, "盐度"=19, "水中油"=20, "高锰酸盐指数"=21, "化学需氧量"=22, "比电导率"=23, "总溶解固体"=24, "pH电极电位"=25] ("下拉列表")
                  n133 = Bundle By Name(cluster=w329, "DO"=1.0) -> (w328:T5)
                  n134 = call "多参数测量数据读取.vi"("探头选择"=w348) -> ("测量数据块"=w327:T6, "添加的数组"=w347:string[][])  [unwired: 8 in, 1 out]
                  n135 = call "多参数测量数据读取.vi"("探头选择"=w332) -> ("测量数据块"=w326:T6, "添加的数组"=w333:string[][])  [unwired: 8 in, 1 out]
                  n136 = global write "多参数全局变量.vi" "DO%数据区"(w327) -> ()
                  n137 = global write "多参数全局变量.vi" "DO数据区"(w326) -> ()
                  n138 = Index Array(array=w347, index (col) #1=1 ("禁用的索引 (列)"), index (col) #2=0 ("禁用的索引 (列)")) -> (element #1=w338:string[], element #2=w341:string[])  [unwired: 2 in]
                  n139 = Index Array(array=w333, index (col)=1 ("禁用的索引 (列)")) -> (element=w337:string[])  [unwired: 1 in]
                  n140 = Insert Into Array(array=w338, index=0 ("索引"), new element="DO_%") -> (w342:string[])
                  n141 = Insert Into Array(array=w337, index=0 ("索引"), new element="DO_mg/L") -> (w331:string[])
                  n142 = Insert Into Array(array=w344, new element #1=w342, new element #2=w331) -> (w343:string[][])  [unwired: 2 in]
                }
                frame 19 {
                  w363 = u16 19 items=["氨氮"=3, "水温"=9, "pH"=10, "溶解氧"=11, "电导率"=12, "浊度"=13, "叶绿素a"=14, "藻密度"=15, "蓝绿藻"=16, "氧化还原电位"=17, "溶解氧%"=18, "盐度"=19, "水中油"=20, "高锰酸盐指数"=21, "化学需氧量"=22, "比电导率"=23, "总溶解固体"=24, "pH电极电位"=25] ("下拉列表")
                  n143 = Bundle By Name(cluster=w351, "Cond"=1.0 ("DO")) -> (w350:T5)
                  n144 = call "多参数测量数据读取.vi"("探头选择"=w363) -> ("测量数据块"=w349:T6, "添加的数组"=w362:string[][])  [unwired: 8 in, 1 out]
                  n145 = global write "多参数全局变量.vi" "Sal数据区"(w349) -> ()
                  n146 = Index Array(array=w362, index (col) #1=1 ("禁用的索引 (列)"), index (col) #2=0 ("禁用的索引 (列)")) -> (element #1=w353:string[], element #2=w356:string[])  [unwired: 2 in]
                  n147 = Insert Into Array(array=w353, index=0 ("索引"), new element="盐度") -> (w357:string[])
                  n148 = Insert Into Array(array=w359, new element=w357) -> (w358:string[][])  [unwired: 2 in]
                }
                frame 20 {
                  w375 = u16 20 items=["氨氮"=3, "水温"=9, "pH"=10, "溶解氧"=11, "电导率"=12, "浊度"=13, "叶绿素a"=14, "藻密度"=15, "蓝绿藻"=16, "氧化还原电位"=17, "溶解氧%"=18, "盐度"=19, "水中油"=20, "高锰酸盐指数"=21, "化学需氧量"=22, "比电导率"=23, "总溶解固体"=24, "pH电极电位"=25] ("下拉列表")
                  n149 = call "多参数测量数据读取.vi"("探头选择"=w375) -> ("添加的数组"=w374:string[][])  [unwired: 8 in, 2 out]
                  n150 = Index Array(array=w374, index (col) #1=1 ("禁用的索引 (列)"), index (col) #2=0 ("禁用的索引 (列)")) -> (element #1=w365:string[], element #2=w368:string[])  [unwired: 2 in]
                  n151 = Insert Into Array(array=w365, index=0 ("索引"), new element="水中油") -> (w369:string[])
                  n152 = Insert Into Array(array=w371, new element=w369) -> (w370:string[][])  [unwired: 2 in]
                }
                frame 21 {
                  w387 = u16 21 items=["氨氮"=3, "水温"=9, "pH"=10, "溶解氧"=11, "电导率"=12, "浊度"=13, "叶绿素a"=14, "藻密度"=15, "蓝绿藻"=16, "氧化还原电位"=17, "溶解氧%"=18, "盐度"=19, "水中油"=20, "高锰酸盐指数"=21, "化学需氧量"=22, "比电导率"=23, "总溶解固体"=24, "pH电极电位"=25] ("下拉列表")
                  n153 = call "多参数测量数据读取.vi"("探头选择"=w387) -> ("添加的数组"=w386:string[][])  [unwired: 8 in, 2 out]
                  n154 = Index Array(array=w386, index (col) #1=1 ("禁用的索引 (列)"), index (col) #2=0 ("禁用的索引 (列)")) -> (element #1=w377:string[], element #2=w380:string[])  [unwired: 2 in]
                  n155 = Insert Into Array(array=w377, index=0 ("索引"), new element="高锰酸盐指数") -> (w381:string[])
                  n156 = Insert Into Array(array=w383, new element=w381) -> (w382:string[][])  [unwired: 2 in]
                }
                frame 22 {
                  w399 = u16 22 items=["氨氮"=3, "水温"=9, "pH"=10, "溶解氧"=11, "电导率"=12, "浊度"=13, "叶绿素a"=14, "藻密度"=15, "蓝绿藻"=16, "氧化还原电位"=17, "溶解氧%"=18, "盐度"=19, "水中油"=20, "高锰酸盐指数"=21, "化学需氧量"=22, "比电导率"=23, "总溶解固体"=24, "pH电极电位"=25] ("下拉列表")
                  n157 = call "多参数测量数据读取.vi"("探头选择"=w399) -> ("添加的数组"=w398:string[][])  [unwired: 8 in, 2 out]
                  n158 = Index Array(array=w398, index (col) #1=1 ("禁用的索引 (列)"), index (col) #2=0 ("禁用的索引 (列)")) -> (element #1=w389:string[], element #2=w392:string[])  [unwired: 2 in]
                  n159 = Insert Into Array(array=w389, index=0 ("索引"), new element="化学需氧量") -> (w393:string[])
                  n160 = Insert Into Array(array=w395, new element=w393) -> (w394:string[][])  [unwired: 2 in]
                }
                frame 23 {
                  w407 = u16 24 items=["氨氮"=3, "水温"=9, "pH"=10, "溶解氧"=11, "电导率"=12, "浊度"=13, "叶绿素a"=14, "藻密度"=15, "蓝绿藻"=16, "氧化还原电位"=17, "溶解氧%"=18, "盐度"=19, "水中油"=20, "高锰酸盐指数"=21, "化学需氧量"=22, "比电导率"=23, "总溶解固体"=24, "pH电极电位"=25] ("下拉列表")
                  w418 = u16 19 items=["氨氮"=3, "水温"=9, "pH"=10, "溶解氧"=11, "电导率"=12, "浊度"=13, "叶绿素a"=14, "藻密度"=15, "蓝绿藻"=16, "氧化还原电位"=17, "溶解氧%"=18, "盐度"=19, "水中油"=20, "高锰酸盐指数"=21, "化学需氧量"=22, "比电导率"=23, "总溶解固体"=24, "pH电极电位"=25] ("下拉列表")
                  w419 = u16 12 items=["氨氮"=3, "水温"=9, "pH"=10, "溶解氧"=11, "电导率"=12, "浊度"=13, "叶绿素a"=14, "藻密度"=15, "蓝绿藻"=16, "氧化还原电位"=17, "溶解氧%"=18, "盐度"=19, "水中油"=20, "高锰酸盐指数"=21, "化学需氧量"=22, "比电导率"=23, "总溶解固体"=24, "pH电极电位"=25] ("下拉列表")
                  w438 = u16 23 items=["氨氮"=3, "水温"=9, "pH"=10, "溶解氧"=11, "电导率"=12, "浊度"=13, "叶绿素a"=14, "藻密度"=15, "蓝绿藻"=16, "氧化还原电位"=17, "溶解氧%"=18, "盐度"=19, "水中油"=20, "高锰酸盐指数"=21, "化学需氧量"=22, "比电导率"=23, "总溶解固体"=24, "pH电极电位"=25] ("下拉列表")
                  n161 = Bundle By Name(cluster=w426, "Cond"=1.0 ("DO")) -> (w425:T5)
                  n162 = call "多参数测量数据读取.vi"("探头选择"=w438) -> ("测量数据块"=w401:T6, "添加的数组"=w437:string[][])  [unwired: 8 in, 1 out]
                  n163 = call "多参数测量数据读取.vi"("探头选择"=w419) -> ("测量数据块"=w403:T6, "添加的数组"=w420:string[][])  [unwired: 8 in, 1 out]
                  n164 = call "多参数测量数据读取.vi"("探头选择"=w418) -> ("测量数据块"=w402:T6, "添加的数组"=w417:string[][])  [unwired: 8 in, 1 out]
                  n165 = call "多参数测量数据读取.vi"("探头选择"=w407) -> ("测量数据块"=w400:T6, "添加的数组"=w408:string[][])  [unwired: 8 in, 1 out]
                  n166 = global write "多参数全局变量.vi" "spCond数据区"(w401) -> ()
                  n167 = global write "多参数全局变量.vi" "Cond数据区"(w403) -> ()
                  n168 = global write "多参数全局变量.vi" "TDS数据区"(w400) -> ()
                  n169 = global write "多参数全局变量.vi" "Sal数据区"(w402) -> ()
                  n170 = Index Array(array=w437, index (col) #1=1 ("禁用的索引 (列)"), index (col) #2=0 ("禁用的索引 (列)")) -> (element #1=w428:string[], element #2=w431:string[])  [unwired: 2 in]
                  n171 = Index Array(array=w420, index (col)=1 ("禁用的索引 (列)")) -> (element=w424:string[])  [unwired: 1 in]
                  n172 = Index Array(array=w417, index (col)=1 ("禁用的索引 (列)")) -> (element=w413:string[])  [unwired: 1 in]
                  n173 = Index Array(array=w408, index (col)=1 ("禁用的索引 (列)")) -> (element=w412:string[])  [unwired: 1 in]
                  n174 = Insert Into Array(array=w412, index=0 ("索引"), new element="TDS") -> (w404:string[])
                  n175 = Insert Into Array(array=w413, index=0 ("索引"), new element="盐度") -> (w405:string[])
                  n176 = Insert Into Array(array=w424, index=0 ("索引"), new element="Cond") -> (w406:string[])
                  n177 = Insert Into Array(array=w428, index=0 ("索引"), new element="spCond") -> (w432:string[])
                  n178 = Insert Into Array(array=w434, new element #1=w432, new element #2=w406, new element #3=w405, new element #4=w404) -> (w433:string[][])  [unwired: 2 in]
                }
                frame 24 {
                  w452 = u16 24 items=["氨氮"=3, "水温"=9, "pH"=10, "溶解氧"=11, "电导率"=12, "浊度"=13, "叶绿素a"=14, "藻密度"=15, "蓝绿藻"=16, "氧化还原电位"=17, "溶解氧%"=18, "盐度"=19, "水中油"=20, "高锰酸盐指数"=21, "化学需氧量"=22, "比电导率"=23, "总溶解固体"=24, "pH电极电位"=25] ("下拉列表")
                  n179 = Bundle By Name(cluster=w440, "Cond"=1.0 ("DO")) -> (w439:T5)
                  n180 = call "多参数测量数据读取.vi"("探头选择"=w452) -> ("添加的数组"=w451:string[][])  [unwired: 8 in, 2 out]
                  n181 = Index Array(array=w451, index (col) #1=1 ("禁用的索引 (列)"), index (col) #2=0 ("禁用的索引 (列)")) -> (element #1=w442:string[], element #2=w445:string[])  [unwired: 2 in]
                  n182 = Insert Into Array(array=w442, index=0 ("索引"), new element="总溶解固体") -> (w446:string[])
                  n183 = Insert Into Array(array=w448, new element=w446) -> (w447:string[][])  [unwired: 2 in]
                }
                frame 25 {
                  w466 = u16 25 items=["氨氮"=3, "水温"=9, "pH"=10, "溶解氧"=11, "电导率"=12, "浊度"=13, "叶绿素a"=14, "藻密度"=15, "蓝绿藻"=16, "氧化还原电位"=17, "溶解氧%"=18, "盐度"=19, "水中油"=20, "高锰酸盐指数"=21, "化学需氧量"=22, "比电导率"=23, "总溶解固体"=24, "pH电极电位"=25] ("下拉列表")
                  n184 = Bundle By Name(cluster=w454, "pH"=1.0 ("DO")) -> (w453:T5)
                  n185 = call "多参数测量数据读取.vi"("探头选择"=w466) -> ("添加的数组"=w465:string[][])  [unwired: 8 in, 2 out]
                  n186 = Index Array(array=w465, index (col) #1=1 ("禁用的索引 (列)"), index (col) #2=0 ("禁用的索引 (列)")) -> (element #1=w456:string[], element #2=w459:string[])  [unwired: 2 in]
                  n187 = Insert Into Array(array=w456, index=0 ("索引"), new element="pH电极电位") -> (w460:string[])
                  n188 = Insert Into Array(array=w462, new element=w460) -> (w461:string[][])  [unwired: 2 in]
                }
              }
            }
            n189 = global write "多参数全局变量.vi" "传感器通道号"(w117) -> ()
            n190 = Insert Into Array(array=w129, index=0 ("索引"), new element="参数名" ("新元素/子数组")) -> (w133:string[])
            n191 = property on="数据区" class="MCListbox (严格)"("ColHdrString"=w133, "ItemNames"=w128) -> ()  [unwired: 2 in, 2 out]
          }
          frame Error {
          }
        }
      }
    }
  }
  n192 = property on="窗格" class="Pane"("Origin"=T2 {"Horizontal"=0, "Vertical"=0} ("原点")) -> ()  [unwired: 2 in, 2 out]
  n193 = property on="打开串口" class="Bool (严格)"("Val(Sgnl)"=TRUE ("值(信号)")) -> (error out=w1:errorcluster)  [unwired: 2 in, 1 out]
  n194 = Obtain Notifier(name (unnamed)="MPFlow" ("名称（未命名）"), notification data type=FALSE) -> (notifier out=w8:refnum<notifier>)  [unwired: 2 in, 2 out]
  n195 = control-ref of="控制命令区探头选择"() -> (w7:refnum<vi>)
  n196 = control-ref of="校准区探头选择"() -> (w4:refnum<vi>)
  n197 = control-ref of="手动通电"() -> (w3:refnum<vi>)
  n198 = control-ref of="K"() -> (w6:refnum<vi>)
  n199 = control-ref of="B"() -> (w5:refnum<vi>)
  n200 = while {
    tunnel: w9 -> [w473]
    tunnel: w8 -> [w472]
    tunnel: w7 -> [w471]
    tunnel: w6 -> [w470]
    tunnel: w5 -> [w469]
    tunnel: w4 -> [w468]
    tunnel: w3 -> [w467]
    tunnel: w1 -> [_]
    stop <- FALSE stop-if-true
    n201 = event shown="[7] \"传感器参数读取\": 值改变" {
      selector: _ -> [_ _ _ _ _ _ _ _ _ _ _ _ _ _ _ _ _ _ _ _ _ _]
      dyn-events: _ -> [_ _ _ _ _ _ _ _ _ _ _ _ _ _ _ _ _ _ _ _ _ _]
      timeout: _ -> [_ _ _ _ _ _ _ _ _ _ _ _ _ _ _ _ _ _ _ _ _ _]
      tunnel: w473 -> [_ _ _ w489 _ _ _ _ _ _ _ _ _ _ _ _ _ _ _ _ _ _]
      tunnel: w472 -> [_ _ _ _ w511 _ _ _ _ _ _ _ _ _ _ _ _ _ _ _ _ _]
      tunnel: w471 -> [_ _ _ _ _ _ _ _ _ _ _ _ _ _ _ w578 w589 _ _ _ _ _]
      tunnel: w470 -> [_ _ _ _ _ _ _ _ _ _ _ _ _ _ _ _ _ w600 _ _ _ _]
      tunnel: w469 -> [_ _ _ _ _ _ _ _ _ _ _ _ _ _ _ _ _ w602 _ _ _ _]
      tunnel: w468 -> [_ _ _ _ _ _ _ _ _ _ _ _ _ _ _ _ _ w604 _ w620 _ _]
      tunnel: w467 -> [_ _ _ _ _ _ _ w519 w524 w529 w535 w540 w549 w558 w567 w576 w587 w598 _ w618 w630 _]
      event Timeout {
        n202 = event-data() -> ()  [unwired: 1 in, 3 out]
      }
      event "释放串口": Value Change {
        n203 = event-data() -> ("NewVal"=w475:bool)  [unwired: 1 in, 5 out]
        n204 = case shown="真" w475 {
          frame False {
          }
          frame True {
            n205 = call "多参数通讯.vi"("STEP"=enum16{"open", "read", "write", "close"}."close") -> ("error out"=w476:errorcluster)  [unwired: 8 in, 2 out]
            n206 = case shown="无错误" w476 {
              frame No Error {
                n207 = property on="打开串口" class="Bool (严格)"("DisabledEnum"=T7."Enabled" ("禁用")) -> ()  [unwired: 2 in, 2 out]
              }
              frame Error {
              }
            }
          }
        }
      }
      event "打开串口": Value Change {
        n208 = event-data() -> ("NewVal"=w479:bool)  [unwired: 1 in, 5 out]
        n209 = case shown="真" w479 {
          frame False {
          }
          frame True {
            n210 = call "多参数通讯.vi"("STEP"=enum16{"open", "read", "write", "close"}."open") -> ("error out"=w480:errorcluster)  [unwired: 8 in, 2 out]
            n211 = case shown="错误" w480 {
              tunnel: [T7."Disabled and Grayed Out" ("禁用") T7."Enabled" ("禁用")] -> w482
              frame No Error {
              }
              frame Error {
                n212 = One Button Dialog(message="多参数串口打开失败" ("消息")) -> ()  [unwired: 1 in, 1 out]
              }
            }
            n213 = property on="打开串口" class="Bool (严格)"("DisabledEnum"=w482, "Value"=FALSE ("打开串口")) -> ()  [unwired: 2 in, 2 out]
          }
        }
      }
      event "手动启动": Value Change {
        n214 = event-data() -> ()  [unwired: 1 in, 6 out]
        n215 = call "多参数启动参数对话框.vi"() -> ("确认"=w488:bool, "测量时间"=w487:dbl)  [unwired: 10 in]
        n216 = case shown="真" w488 {
          tunnel: w489 -> [_ w491]
          tunnel: w487 -> [_ w490]
          frame False {
          }
          frame True {
            n217 = property class="VI"(reference=w491) -> ("Name"=w495:string, "Exec.State"=w493:T11)  [unwired: 1 in, 2 out]
            n218 = Open VI Reference(type specifier VI Refnum (for type only)=refnum<vi> refnum ("类型说明符VI引用句柄（仅用于类型）"), vi path=w495, options=128 ("选项")) -> (vi reference=w494:refnum<vi>)  [unwired: 3 in, 1 out]
            n219 = case shown="\"Idle\"" w493 {
              tunnel: w494 -> [w499 w506]
              tunnel: [w499 w505] -> w492
              tunnel: w490 -> [_ w500]
              frame "Bad", Default {
                n220 = One Button Dialog(message="仪器已经启动，无需重复启动" ("消息")) -> ()  [unwired: 1 in, 1 out]
              }
              frame "Idle" {
                n221 = global read "系统变量.vi" "运行模式"() -> (w502:enum16{"维护模式", "常规模式", "应急模式", "质控模式"})
                n222 = case shown="\"常规模式\", 默认" w502 {
                  tunnel: ["M" ("数据标记表") "hd" ("数据标记表")] -> w501
                  frame "维护模式" {
                  }
                  frame "常规模式", Default {
                  }
                }
                n223 = Bundle By Name(cluster=T8 {"测量模式"=enum."水样测试", "数据标记表"="", "测量时间"=0.0} ("启动参数"), "数据标记表"=w501, "测量时间"=w500) -> (w503:T8)
                n224 = call-by-ref "开始异步调用"(reference=w506, "启动参数"=w503) -> (reference out=w505:refnum<vi>)  [unwired: 12 in, 1 out]
              }
            }
            n225 = Close Reference(reference=w492) -> ()  [unwired: 1 in, 1 out]
          }
        }
      }
      event "停止": Value Change {
        n226 = event-data() -> ()  [unwired: 1 in, 6 out]
        n227 = Two Button Dialog(message="请再一次确认是否停止测量" ("消息")) -> (T button?=w509:bool)  [unwired: 2 in]
        n228 = case shown="真" w509 {
          tunnel: w511 -> [_ w514]
          frame False {
          }
          frame True {
            w512 = u16 11 items=["启动测量（全部）"=1, "初始化（清洗）"=10, "停止测量（全部）"=11, "校时"=13, "启动测量（单个传感器）"=19, "停止测量（单个传感器）"=20] ("控制命令")
            w513 = u16 10 items=["氨氮"=3, "水温"=9, "pH值"=10, "溶解氧"=11, "电导率"=12, "浊度"=13, "叶绿素a"=14, "藻密度"=15, "蓝绿藻"=16, "氧化还原电位"=17, "溶解氧%"=18, "盐度"=19] ("站号")
            n229 = Send Notification(notification=TRUE ("通知"), notifier=w514) -> ()  [unwired: 1 in, 2 out]
            n230 = call "多参数控制命令.vi"("控制命令"=w512, "站号"=w513) -> ()  [unwired: 9 in, 1 out]
          }
        }
      }
      event "设置": Value Change {
        n231 = event-data() -> ()  [unwired: 1 in, 6 out]
        n232 = property on="窗格" class="Pane"("Origin"=T2 {"Horizontal"=0, "Vertical"=528} ("原点")) -> ()  [unwired: 2 in, 2 out]
      }
      event "返回": Value Change {
        n233 = event-data() -> ()  [unwired: 1 in, 6 out]
        n234 = property on="窗格" class="Pane"("Origin"=T2 {"Horizontal"=0, "Vertical"=0} ("原点")) -> ()  [unwired: 2 in, 2 out]
      }
      event "传感器参数读取": Value Change {
        n235 = event-data() -> ()  [unwired: 1 in, 6 out]
        n236 = property class="Bool (严格)"(reference=w519) -> ("Value"=w518:bool)  [unwired: 1 in, 2 out]
        n237 = case shown="真" w518 {
          frame False {
            n238 = One Button Dialog(message="启动失败，请先通电" ("消息")) -> ()  [unwired: 1 in, 1 out]
          }
          frame True {
            n239 = call "多参数传感器参数读取.vi"() -> ("error out"=w521:errorcluster, "添加的数组"=w522:string[][])  [unwired: 10 in]
            n240 = call <vilib>:"General Error Handler.vi"("error in (no error)"=w521) -> ()  [unwired: 10 in, 5 out]
            n241 = property on="传感器区" class="MCListbox (严格)"("ItemNames"=w522) -> ()  [unwired: 2 in, 2 out]
          }
        }
      }
      event "关键参数区读取": Value Change {
        n242 = event-data() -> ()  [unwired: 1 in, 6 out]
        n243 = property class="Bool (严格)"(reference=w524) -> ("Value"=w523:bool)  [unwired: 1 in, 2 out]
        n244 = case shown="假" w523 {
          frame False {
            n245 = One Button Dialog(message="启动失败，请先通电" ("消息")) -> ()  [unwired: 1 in, 1 out]
          }
          frame True {
            n246 = call "多参数关键参数读取.vi"() -> ("error out"=w526:errorcluster, "添加的数组"=w527:string[][])  [unwired: 10 in]
            n247 = call <vilib>:"General Error Handler.vi"("error in (no error)"=w526) -> ()  [unwired: 10 in, 5 out]
            n248 = property on="关键参数区" class="MCListbox (严格)"("ItemNames"=w527) -> ()  [unwired: 2 in, 2 out]
          }
        }
      }
      event "测量数据区读取": Value Change {
        n249 = event-data() -> ()  [unwired: 1 in, 6 out]
        n250 = property class="Bool (严格)"(reference=w529) -> ("Value"=w528:bool)  [unwired: 1 in, 2 out]
        n251 = case shown="假" w528 {
          frame False {
            n252 = One Button Dialog(message="启动失败，请先通电" ("消息")) -> ()  [unwired: 1 in, 1 out]
          }
          frame True {
            n253 = call "多参数测量数据读取.vi"("探头选择"="探头选择") -> ("error out"=w532:errorcluster, "添加的数组"=w533:string[][])  [unwired: 8 in, 1 out]
            n254 = call <vilib>:"General Error Handler.vi"("error in (no error)"=w532) -> ()  [unwired: 10 in, 5 out]
            n255 = property on="测量数据区" class="MCListbox (严格)"("ItemNames"=w533) -> ()  [unwired: 2 in, 2 out]
          }
        }
      }
      event "状态告警区读取": Value Change {
        n256 = event-data() -> ()  [unwired: 1 in, 6 out]
        n257 = property class="Bool (严格)"(reference=w535) -> ("Value"=w534:bool)  [unwired: 1 in, 2 out]
        n258 = case shown="真" w534 {
          frame False {
            n259 = One Button Dialog(message="启动失败，请先通电" ("消息")) -> ()  [unwired: 1 in, 1 out]
          }
          frame True {
            n260 = call "多参数状态告警区读取.vi"() -> ("error out"=w537:errorcluster, "添加的数组"=w538:string[][])  [unwired: 9 in, 1 out]
            n261 = call <vilib>:"General Error Handler.vi"("error in (no error)"=w537) -> ()  [unwired: 10 in, 5 out]
            n262 = property on="状态告警区" class="MCListbox (严格)"("ItemNames"=w538) -> ()  [unwired: 2 in, 2 out]
          }
        }
      }
      event "同步时间": Value Change {
        n263 = event-data() -> ()  [unwired: 1 in, 6 out]
        n264 = property class="Bool (严格)"(reference=w540) -> ("Value"=w539:bool)  [unwired: 1 in, 2 out]
        n265 = case shown="假" w539 {
          frame False {
            n266 = One Button Dialog(message="启动失败，请先通电" ("消息")) -> ()  [unwired: 1 in, 1 out]
          }
          frame True {
            w542 = u16 13 items=["启动测量（全部）"=1, "初始化（清洗）"=10, "停止测量（全部）"=11, "校时"=13, "启动测量（单个传感器）"=19, "停止测量（单个传感器）"=20] ("控制命令")
            w543 = u16 9 items=["氨氮"=3, "水温"=9, "pH值"=10, "溶解氧"=11, "电导率"=12, "浊度"=13, "叶绿素a"=14, "藻密度"=15, "蓝绿藻"=16, "氧化还原电位"=17, "溶解氧%"=18, "盐度"=19] ("站号")
            n267 = call "多参数控制命令.vi"("控制命令"=w542, "站号"=w543) -> ("error out"=w545:errorcluster)  [unwired: 9 in]
            n268 = case shown="错误" w545 {
              tunnel: ["时间同步成功" ("消息") "时间同步失败" ("消息")] -> w544
              frame No Error {
              }
              frame Error {
              }
            }
            n269 = One Button Dialog(message=w544) -> ()  [unwired: 1 in, 1 out]
          }
        }
      }
      event "启动测量(全部)": Value Change {
        n270 = event-data() -> ()  [unwired: 1 in, 6 out]
        n271 = property class="Bool (严格)"(reference=w549) -> ("Value"=w548:bool)  [unwired: 1 in, 2 out]
        n272 = case shown="假" w548 {
          frame False {
            n273 = One Button Dialog(message="启动失败，请先通电" ("消息")) -> ()  [unwired: 1 in, 1 out]
          }
          frame True {
            w551 = u16 1 items=["启动测量（全部）"=1, "初始化（清洗）"=10, "停止测量（全部）"=11, "校时"=13, "启动测量（单个传感器）"=19, "停止测量（单个传感器）"=20] ("控制命令")
            w552 = u16 9 items=["氨氮"=3, "水温"=9, "pH值"=10, "溶解氧"=11, "电导率"=12, "浊度"=13, "叶绿素a"=14, "藻密度"=15, "蓝绿藻"=16, "氧化还原电位"=17, "溶解氧%"=18, "盐度"=19] ("站号")
            n274 = call "多参数控制命令.vi"("控制命令"=w551, "站号"=w552) -> ("error out"=w554:errorcluster)  [unwired: 9 in]
            n275 = case shown="无错误" w554 {
              tunnel: ["启动成功" ("消息") "启动失败" ("消息")] -> w553
              frame No Error {
              }
              frame Error {
              }
            }
            n276 = One Button Dialog(message=w553) -> ()  [unwired: 1 in, 1 out]
          }
        }
      }
      event "停止测量(全部)": Value Change {
        n277 = event-data() -> ()  [unwired: 1 in, 6 out]
        n278 = property class="Bool (严格)"(reference=w558) -> ("Value"=w557:bool)  [unwired: 1 in, 2 out]
        n279 = case shown="真" w557 {
          frame False {
            n280 = One Button Dialog(message="启动失败，请先通电" ("消息")) -> ()  [unwired: 1 in, 1 out]
          }
          frame True {
            w562 = u16 11 items=["启动测量（全部）"=1, "初始化（清洗）"=10, "停止测量（全部）"=11, "校时"=13, "启动测量（单个传感器）"=19, "停止测量（单个传感器）"=20] ("控制命令")
            w563 = u16 9 items=["氨氮"=3, "水温"=9, "pH值"=10, "溶解氧"=11, "电导率"=12, "浊度"=13, "叶绿素a"=14, "藻密度"=15, "蓝绿藻"=16, "氧化还原电位"=17, "溶解氧%"=18, "盐度"=19] ("站号")
            n281 = call "多参数控制命令.vi"("控制命令"=w562, "站号"=w563) -> ("error out"=w561:errorcluster)  [unwired: 9 in]
            n282 = case shown="错误" w561 {
              tunnel: ["停止成功" ("消息") "停止失败" ("消息")] -> w560
              frame No Error {
              }
              frame Error {
              }
            }
            n283 = One Button Dialog(message=w560) -> ()  [unwired: 1 in, 1 out]
          }
        }
      }
      event "初始化(清洗)": Value Change {
        n284 = event-data() -> ()  [unwired: 1 in, 6 out]
        n285 = property class="Bool (严格)"(reference=w567) -> ("Value"=w566:bool)  [unwired: 1 in, 2 out]
        n286 = case shown="真" w566 {
          frame False {
            n287 = One Button Dialog(message="启动失败，请先通电" ("消息")) -> ()  [unwired: 1 in, 1 out]
          }
          frame True {
            w571 = u16 10 items=["启动测量（全部）"=1, "初始化（清洗）"=10, "停止测量（全部）"=11, "校时"=13, "启动测量（单个传感器）"=19, "停止测量（单个传感器）"=20] ("控制命令")
            w572 = u16 9 items=["氨氮"=3, "水温"=9, "pH值"=10, "溶解氧"=11, "电导率"=12, "浊度"=13, "叶绿素a"=14, "藻密度"=15, "蓝绿藻"=16, "氧化还原电位"=17, "溶解氧%"=18, "盐度"=19] ("站号")
            n288 = call "多参数控制命令.vi"("控制命令"=w571, "站号"=w572) -> ("error out"=w569:errorcluster)  [unwired: 9 in]
            n289 = case shown="错误" w569 {
              tunnel: ["初始化成功" ("消息") "初始化失败" ("消息")] -> w570
              frame No Error {
              }
              frame Error {
              }
            }
            n290 = One Button Dialog(message=w570) -> ()  [unwired: 1 in, 1 out]
          }
        }
      }
      event "启动测量(单探)": Value Change {
        n291 = event-data() -> ()  [unwired: 1 in, 6 out]
        n292 = property class="Bool (严格)"(reference=w576) -> ("Value"=w575:bool)  [unwired: 1 in, 2 out]
        n293 = property class="Ring (严格)"(reference=w578) -> ("Value"=w577:u16)  [unwired: 1 in, 2 out]
        n294 = case shown="真" w575 {
          tunnel: w577 -> [_ w580]
          frame False {
            n295 = One Button Dialog(message="启动失败，请先通电" ("消息")) -> ()  [unwired: 1 in, 1 out]
          }
          frame True {
            w581 = u16 19 items=["启动测量（全部）"=1, "初始化（清洗）"=10, "停止测量（全部）"=11, "校时"=13, "启动测量（单个传感器）"=19, "停止测量（单个传感器）"=20] ("控制命令")
            n296 = call "多参数控制命令.vi"("控制命令"=w581, "站号"=w580) -> ("error out"=w583:errorcluster)  [unwired: 9 in]
            n297 = case shown="无错误" w583 {
              tunnel: ["启动成功" ("消息") "启动失败" ("消息")] -> w582
              frame No Error {
              }
              frame Error {
              }
            }
            n298 = One Button Dialog(message=w582) -> ()  [unwired: 1 in, 1 out]
          }
        }
      }
      event "停止测量(单探)": Value Change {
        n299 = event-data() -> ()  [unwired: 1 in, 6 out]
        n300 = property class="Bool (严格)"(reference=w587) -> ("Value"=w586:bool)  [unwired: 1 in, 2 out]
        n301 = property class="Ring (严格)"(reference=w589) -> ("Value"=w588:u16)  [unwired: 1 in, 2 out]
        n302 = case shown="真" w586 {
          tunnel: w588 -> [_ w591]
          frame False {
            n303 = One Button Dialog(message="启动失败，请先通电" ("消息")) -> ()  [unwired: 1 in, 1 out]
          }
          frame True {
            w592 = u16 20 items=["启动测量（全部）"=1, "初始化（清洗）"=10, "停止测量（全部）"=11, "校时"=13, "启动测量（单个传感器）"=19, "停止测量（单个传感器）"=20] ("控制命令")
            n304 = call "多参数控制命令.vi"("控制命令"=w592, "站号"=w591) -> ("error out"=w594:errorcluster)  [unwired: 9 in]
            n305 = case shown="错误" w594 {
              tunnel: ["停止成功" ("消息") "停止失败" ("消息")] -> w593
              frame No Error {
              }
              frame Error {
              }
            }
            n306 = One Button Dialog(message=w593) -> ()  [unwired: 1 in, 1 out]
          }
        }
      }
      event "写入KB": Value Change {
        n307 = event-data() -> ()  [unwired: 1 in, 6 out]
        n308 = property class="DigNum (严格)"(reference=w600) -> ("Value"=w599:dbl)  [unwired: 1 in, 2 out]
        n309 = property class="DigNum (严格)"(reference=w602) -> ("Value"=w601:dbl)  [unwired: 1 in, 2 out]
        n310 = property class="Bool (严格)"(reference=w598) -> ("Value"=w597:bool)  [unwired: 1 in, 2 out]
        n311 = property class="Ring (严格)"(reference=w604) -> ("Value"=w603:u16)  [unwired: 1 in, 2 out]
        n312 = case shown="假" w597 {
          tunnel: w603 -> [_ w610]
          tunnel: w601 -> [_ w609]
          tunnel: w599 -> [_ w608]
          frame False {
            n313 = One Button Dialog(message="启动失败，请先通电" ("消息")) -> ()  [unwired: 1 in, 1 out]
          }
          frame True {
            n314 = call "多参数校准写入.vi"("B"=w609, "K"=w608, "站号"=w610) -> ("error out"=w606:errorcluster)  [unwired: 8 in]
            n315 = case shown="错误" w606 {
              tunnel: ["写入成功" ("消息") "写入失败" ("消息")] -> w607
              frame No Error {
              }
              frame Error {
              }
            }
            n316 = One Button Dialog(message=w607) -> ()  [unwired: 1 in, 1 out]
          }
        }
      }
      event "K", "B": Mouse Down {
        n317 = event-data() -> ("CtlRef"=w616:refnum<vi>)  [unwired: 1 in, 5 out]
        n318 = property class="DigNum (严格)"(reference=w616) -> (reference out=w615:refnum<vi>, "Value"=w614:dbl)  [unwired: 1 in, 1 out]
        n319 = call "数字键盘.vi"("OldNumber"=w614) -> ("NewNumber"=w613:sgl)
        n320 = property class="DigNum (严格)"(reference=w615, "Value"=w613) -> ()  [unwired: 1 in, 2 out]
      }
      event "读取KB": Value Change {
        n321 = event-data() -> ()  [unwired: 1 in, 6 out]
        n322 = property class="Bool (严格)"(reference=w618) -> ("Value"=w617:bool)  [unwired: 1 in, 2 out]
        n323 = property class="Ring (严格)"(reference=w620) -> ("Value"=w619:u16)  [unwired: 1 in, 2 out]
        n324 = case shown="真" w617 {
          tunnel: w619 -> [_ w624]
          frame False {
            n325 = One Button Dialog(message="启动失败，请先通电" ("消息")) -> ()  [unwired: 1 in, 1 out]
          }
          frame True {
            n326 = call "多参校准读取.vi"("站号"=w624) -> ("error out"=w622:errorcluster, "B"=→"B":dbl, "K"=→"K":dbl)  [unwired: 8 in]
            n327 = case shown="无错误" w622 {
              tunnel: ["读取成功" ("消息") "读取失败" ("消息")] -> w623
              frame No Error {
              }
              frame Error {
              }
            }
            n328 = One Button Dialog(message=w623) -> ()  [unwired: 1 in, 1 out]
          }
        }
      }
      event "自动校准": Value Change {
        n329 = event-data() -> ()  [unwired: 1 in, 6 out]
        n330 = property class="Bool (严格)"(reference=w630) -> ("Value"=w629:bool)  [unwired: 1 in, 2 out]
        n331 = case shown="真" w629 {
          frame False {
            n332 = One Button Dialog(message="启动失败，请先通电" ("消息")) -> ()  [unwired: 1 in, 1 out]
          }
          frame True {
            n333 = call "多参校准.vi"() -> ()  [unwired: 12 in]
          }
        }
      }
      event "手动通电": Value Change {
        n334 = event-data() -> ("NewVal"=w633:bool)  [unwired: 1 in, 5 out]
        n335 = Boolean To (0,1)(Boolean=w633) -> (0, 1=w632:i16)
        n336 = Bundle By Name(cluster=T9 {"starting address"=0, "holding register value"=0}, "starting address"=u16 302, "holding register value"=w632) -> (w635:T9)
        n337 = call "采配水通讯指令.vi"("数据"=w635, "命令"=T10."单个写入") -> ()  [unwired: 10 in]
      }
    }
  }
